vi "Print.vi"(8 "error in":errorcluster, 11 "Object Type Base in":refnum<class "Object Type Base.lvclass">) -> (0 "error out":errorcluster, 2 "Fields":map{string, string}(c390), 3 "Object Type Base out":refnum<class "Object Type Base.lvclass">)   [LabVIEW 2020, in "Electronic Datasheet.lvlib" / "Object Type Base.lvclass"]
uses:
  Object Type Base.lvclass
  Object Type Base.lvclass/Object Type Base.ctl
  Object Type.ctl
  Electronic Datasheet.lvlib
panel:
  out "DataType":u16(ring) items=["BOOLEAN"=1, "INTEGER8"=2, "INTEGER16"=3, "INTEGER32"=4, "UNSIGNED8"=5, "UNSIGNED16"=6, "UNSIGNED32"=7, "REAL32"=8, "VISIBLE_STRING"=9, "OCTET_STRING"=10, "UNICODE_STRING"=11, "TIME_OF_DAY"=12, "TIME_DIFFERENCE"=13, "RESERVED1"=14, "DOMAIN"=15, "INTEGER24"=16, "REAL64"=17, "INTEGER40"=18, "INTEGER48"=19, "INTEGER56"=20, "INTEGER64"=21, "UNSIGNED24"=22, "RESERVED2"=23, "UNSIGNED40"=24, "UNSIGNED48"=25, "UNSIGNED56"=26, "UNSIGNED64"=27, "RESERVED3"=28, "RESERVED4"=29, "RESERVED5"=30, "RESERVED6"=31, "PDO_COMMUNICATION_PARAMETER"=32, "PDO_MAPPING"=33, "SDO_PARAMETER"=34, "IDENTITY"=35, "RESERVED7"=36]
  out "ObjectType":T1 items=["NULL"=0, "DOMAIN"=2, "DEFTYPE"=5, "DEFSTRUCT"=6, "VAR"=7, "ARRAY"=8, "RECORD"=9]
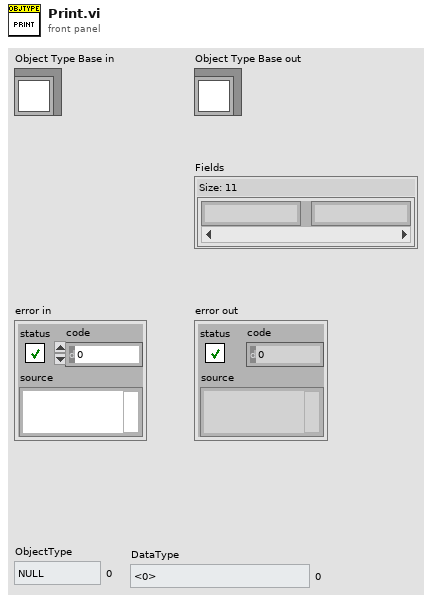
[diagram p1: front panel]
types:
  T1 = typedef "Electronic Datasheet.lvlib/Object Type.ctl" = u8
  T2 = typedef "Electronic Datasheet.lvlib/Access Type.ctl" = enum16{"ro", "wo", "rw", "rwr", "rww", "const"}
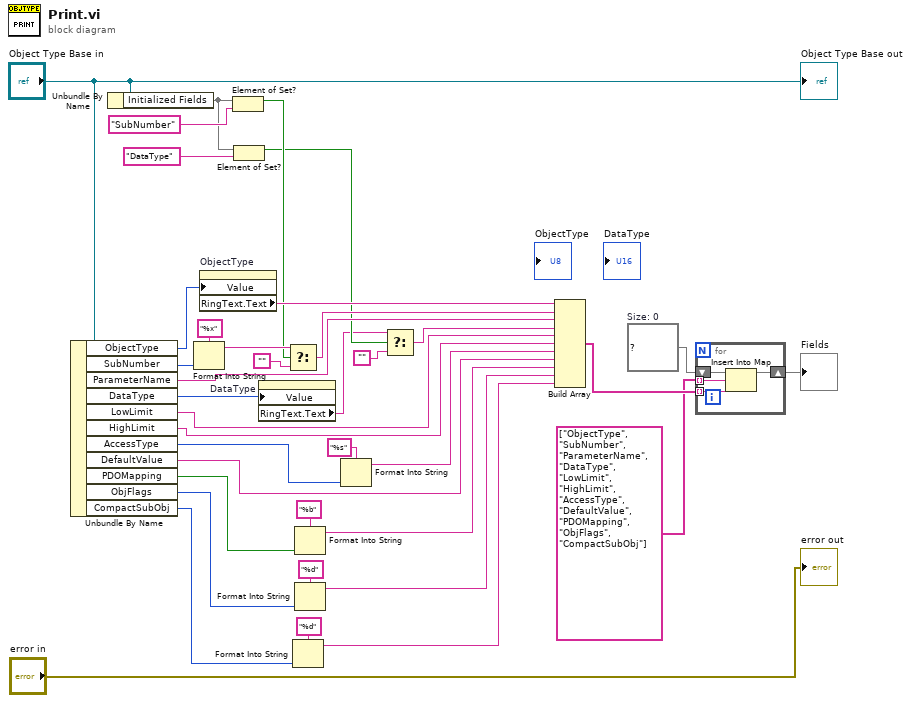
[diagram p0: block diagram]
diagram:
  w33 = map{string, string} {}  # Size: 0
  n1 = Unbundle By Name("Object Type Base in") -> ("ObjectType"=w38:T1, "SubNumber"=w37:u8, "ParameterName"=w30:string, "DataType"=w2:u16, "LowLimit"=w29:string, "HighLimit"=w28:string, "AccessType"=w5:T2, "DefaultValue"=w27:string, "PDOMapping"=w25:bool, "ObjFlags"=w34:u32, "CompactSubObj"=w21:u8)
  n2 = Unbundle By Name("Object Type Base in") -> ("Initialized Fields"=w10:set{string})
  n3 = Format Into String(format string="%x", w37) -> (resulting string=w31:string)  [unwired: 2 in, 1 out]
  n4 = property on="ObjectType" class="Ring (strict)"("Value"=w38) -> ("RingText.Text"=w32:string)  [unwired: 2 in, 2 out]
  n5 = Element of Set?(10:"SubNumber" ("element"), 11:w10) -> (3:w12:bool)
  n6 = Element of Set?(10:"DataType" ("element"), 11:w10) -> (3:w7:bool)
  n7 = property on="DataType" class="Ring (strict)"("Value"=w2) -> ("RingText.Text"=w1:string)  [unwired: 2 in, 2 out]
  n8 = Select(t=w31, s=w12, f="") -> (s? t:f=w13:string)
  n9 = Format Into String(format string="%d", w21) -> (resulting string=w20:string)  [unwired: 2 in, 1 out]
  n10 = Format Into String(format string="%b", w25) -> (resulting string=w24:string)  [unwired: 2 in, 1 out]
  n11 = Format Into String(format string="%d", w34) -> (resulting string=w23:string)  [unwired: 2 in, 1 out]
  n12 = Format Into String(format string="%s", w5) -> (resulting string=w4:string)  [unwired: 2 in, 1 out]
  n13 = Select(t=w1, s=w7, f="") -> (s? t:f=w8:string)
  n14 = Build Array(w32, w13, w30, w8, w29, w28, w4, w27, w24, w23, w20) -> (w19:string[])
  n15 = for {
    shift-right: [w41] -> w18
    shift-left: w33 -> [w42]
    tunnel: string[] ["ObjectType", "SubNumber", "ParameterName", "DataType", "LowLimit", "HighLimit", "AccessType", "DefaultValue", "PDOMapping", "ObjFlags", "CompactSubObj"] -> [w40] mode=indexing
    tunnel: w19 -> [w39] mode=indexing
    n16 = Insert Into Map(map in=w42, key=w40, value=w39) -> (map out=w41:map{string, string})  [unwired: 2 out]
  }
  "Fields" <- w18
  "error out" <- "error in"
  "Object Type Base out" <- "Object Type Base in"
